vi "Write Key (Boolean).vi"(7 "section":string, 8 "error in (no error)":errorcluster, 9 "value":bool, 10 "key":string, 11 "refnum":T1) -> (0 "error out":errorcluster, 2 "found?":bool, 3 "refnum out":T1)   [LabVIEW 2020, in "NI_LVConfig.lvlib"]
doc: "Writes a value to a key in a specified section of the configuration data identified by <B>refnum</B>. This VI modifies data in memory. To write data to disk, use the Close Config Data VI. Wire data to the <B>value</B> input to determine the polymorphic instance to use or manually select the instance."
uses:
  <vilib>/Utility/config.llb/NI_LVConfig.lvlib
  <vilib>/Utility/config.llb/Config Data RefNum.ctl
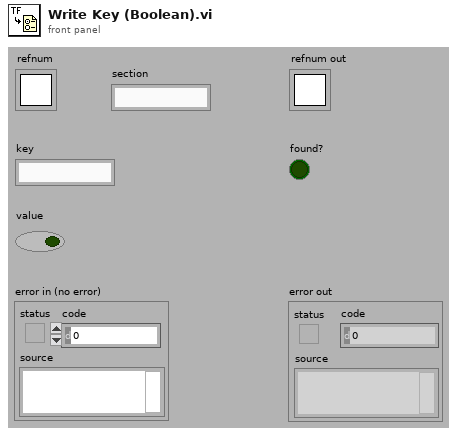
[diagram p1: front panel]
types:
  T1 = typedef "NI_LVConfig.lvlib/Config Data RefNum.ctl" = refnum<k1>
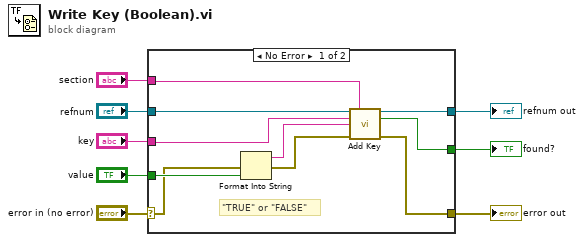
[diagram p0: block diagram]
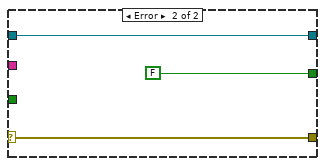
[diagram p2: hidden frame]
diagram:
  n1 = case shown="No Error" "error in (no error)" {
    selector: "error in (no error)" -> [w11 w21]
    tunnel: [w12 w21] -> w7
    tunnel: "section" -> [w14 _]
    tunnel: "key" -> [w17 _]
    tunnel: "value" -> [w18 _]
    tunnel: [w13 FALSE ("key exists?")] -> w3
    tunnel: "refnum" -> [w10 w19]
    tunnel: [w9 w19] -> w1
    frame No Error {
      # "\"TRUE\" or \"FALSE\""
      n2 = Format Into String(error in=w11, w18) -> (resulting string=w15:string, error out=w16:errorcluster)  [unwired: 2 in]
      n3 = call <vilib>:"Add Key.vi"("refnum"=w10, "section"=w14, "key"=w17, "value"=w15, "error in (no error)"=w16) -> ("refnum out"=w9:T1, "key exists?"=w13:bool, "error out"=w12:errorcluster)  [unwired: 1 in, 7 out]
    }
    frame Error {
    }
  }
  "error out" <- w7
  "found?" <- w3
  "refnum out" <- w1
